vi "fa.vi"(7 "fbeta":dbl, 9 "Constants and System Parameters":T1, 10 "Ankle Angle":dbl) -> (2 "fa":dbl)   [LabVIEW 2018]
uses:
  Constants and System Parameters.ctl
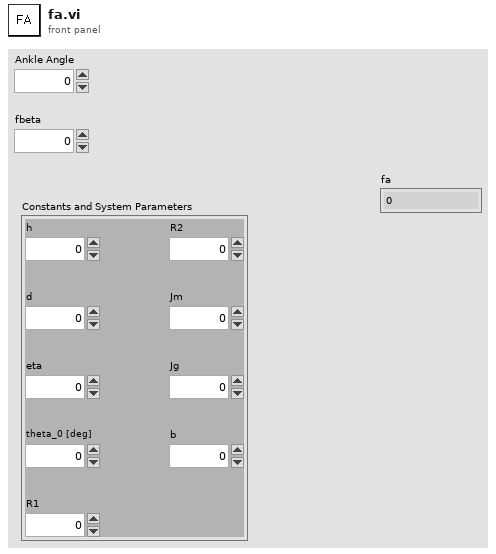
[diagram p1: front panel]
types:
  T1 = typedef "Constants and System Parameters.ctl" = cluster{"h":dbl, "d":dbl, "eta":dbl, "theta_0 [deg]":dbl, "R1":dbl, "R2":dbl, "Jm":dbl, "Jg":dbl, "b":dbl}
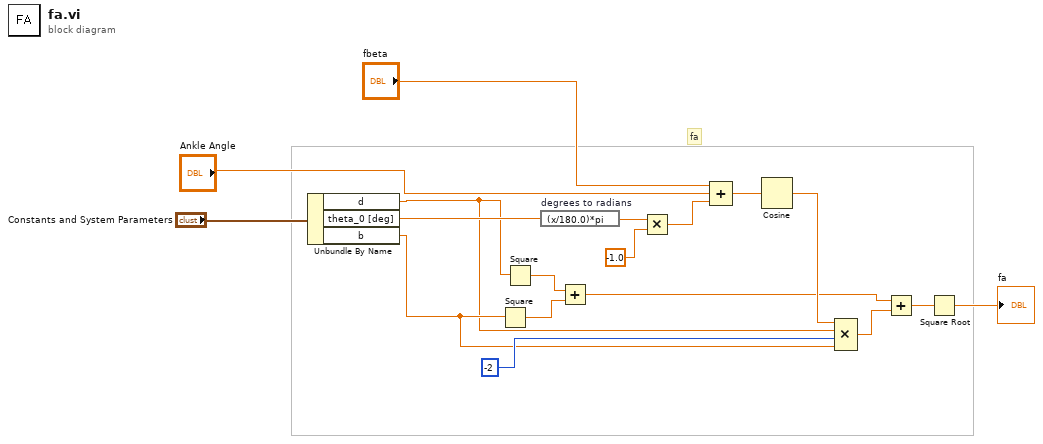
[diagram p0: block diagram]
diagram:
  # "fa"
  n1 = Unbundle By Name("Constants and System Parameters") -> ("d"=w9:dbl, "theta_0 [deg]"=w15:dbl, "b"=w10:dbl)
  n2 = Square(x=w10) -> (x^2=w17:dbl)
  n3 = Square(x=w9) -> (x^2=w18:dbl)
  n4 = expression code="(x/180.0)*pi" "degrees to radians"(w15) -> (w14:dbl)
  n5 = Add(x=w18, y=w17) -> (x+y=w7:dbl)
  n6 = Multiply(x=w14, y=-1.0) -> (x*y=w13:dbl)
  n7 = Compound Arithmetic op=ADD("fbeta", "Ankle Angle", w13) -> (w11:dbl)
  n8 = Cosine(x=w11) -> (cos(x)=w8:dbl)
  n9 = Compound Arithmetic op=MULTIPLY(w8, w9, -2, w10) -> (w6:dbl)
  n10 = Add(x=w7, y=w6) -> (x+y=w5:dbl)
  n11 = Square Root(x=w5) -> (sqrt(x)=→"fa":dbl)
